vi "set channel.vi"(8 "error in":errorcluster, 10 "channel":refnum<class "TBM channel.lvclass">, 11 "Scan Engine configuration in":refnum<class "Scan Engine configuration.lvclass">) -> (0 "error out":errorcluster, 3 "Scan Engine configuration out":refnum<class "Scan Engine configuration.lvclass">)   [LabVIEW 2013, in "Scan Engine configuration.lvclass"]
uses:
  Scan Engine configuration.lvclass
  <vilib>/NI/Tag Bus Module Framework/channel/TBM channel.lvclass
  <vilib>/NI/Tag Bus/tag/tag descriptor.lvclass/tag descriptor.ctl
  Scan Engine configuration.lvclass/Scan Engine configuration.ctl
  <vilib>/NI/Tag Bus/tag/tag descriptor.lvclass
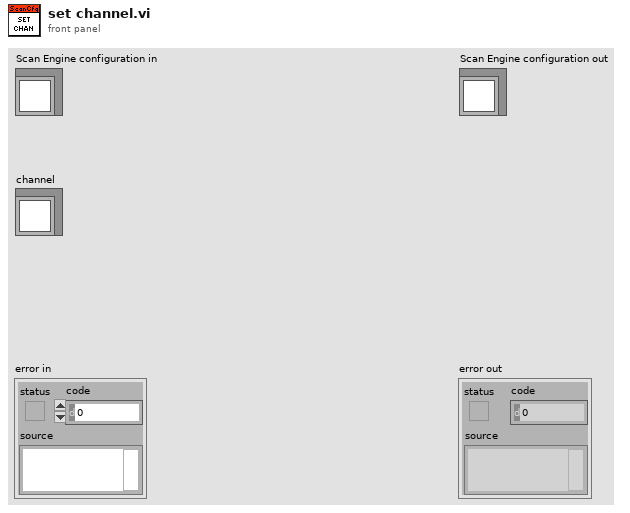
[diagram p1: front panel]
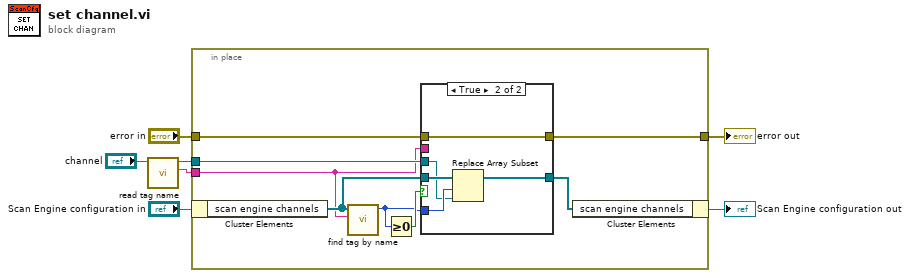
[diagram p0: block diagram]
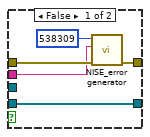
[diagram p2: hidden frame]
diagram:
  n1 = call <vilib>:"read tag name.vi"("system tag in"="channel") -> ("name"=w6:string, "system tag out"=w7:refnum<class "TBM channel.lvclass">)  [unwired: 8 in, 1 out]
  n2 = in-place {
    in-place-border: [w14] -> w2
    in-place-border: "error in" -> [w12]
    in-place-border: w7 -> [w11]
    in-place-border: w6 -> [w10]
    n3 = in-place-cluster #1("Scan Engine configuration in") -> ("scan engine channels"=w15:refnum<class "TBM channel.lvclass">[])
    n4 = call <vilib>:"find tag by name.vi"("name"=w10, "tags in"=w15) -> ("index"=w8:i32)  [unwired: 9 in]
    n5 = Greater Or Equal To 0?(x=w8) -> (x >= 0?=w9:bool)
    n6 = case shown="True" w9 {
      tunnel: w8 -> [_ w22]
      tunnel: w15 -> [w18 w24]
      tunnel: [w19 w25] -> w14
      tunnel: [w18 w23] -> w13
      tunnel: w12 -> [w17 w25]
      tunnel: w11 -> [_ w21]
      tunnel: w10 -> [w16 _]
      frame False {
        n7 = call <vilib>:"NISE_error generator.vi"("error in"=w17, "append error message"=w16, "error code (0)"=538309) -> ("error out"=w19:errorcluster)  [unwired: 6 in]
      }
      frame True {
        n8 = Replace Array Subset(array=w24, new element=w21, index=w22) -> (w23:refnum<class "TBM channel.lvclass">[])
      }
    }
    n9 = in-place-cluster #1("scan engine channels"=w13) -> (→"Scan Engine configuration out":refnum<class "Scan Engine configuration.lvclass">)
  }
  "error out" <- w2
